vi "UE9 Multiple AIN and Multiple LabJack Loop Example.vi"() -> ()   [LabVIEW 2021]
panel:
  in  "stop":bool
  in  "Ranges B":string[](array[string])=["LJ_rgBIP5V", "LJ_rgBIP5V"]
  in  "Channels B":i32[](array[numeric])=[0, 1]
  out "Values Read B":dbl[](array[numeric]) format="%.6f"
  in  "Address B":string="3"
  in  "ConnectionType":string="LJ_ctUSB"
  in  "Address A":string="2"
  in  "Ranges A":string[](array[string])=["LJ_rgBIP5V", "LJ_rgBIP5V"]
  in  "Channels A":i32[](array[numeric])=[0, 1]
  out "Values Read A":dbl[](array[numeric]) format="%.6f"
  out "Error Message":string
  in  "Resolution":i32=17
  in  "error in":errorcluster
  out "error out":errorcluster
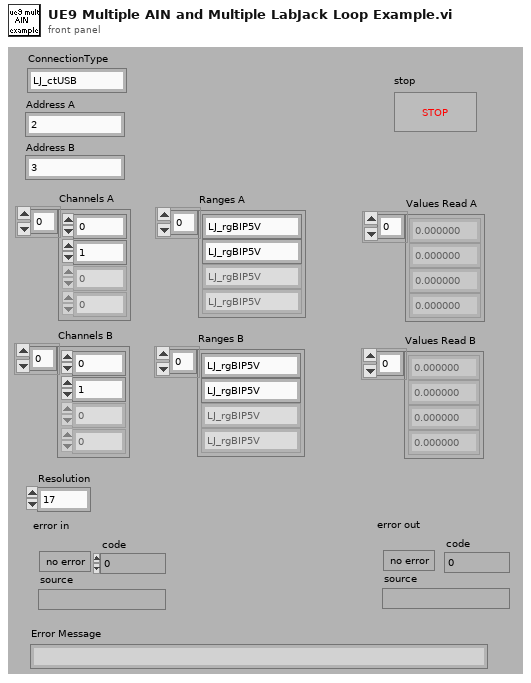
[diagram p1: front panel]
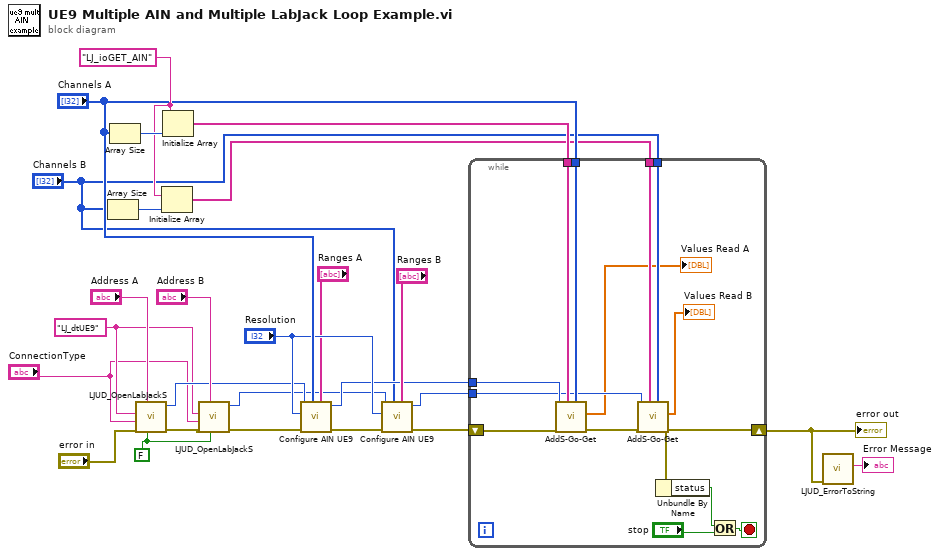
[diagram p0: block diagram]
diagram:
  w2 = "LJ_dtUE9"
  w21 = "LJ_ioGET_AIN" ("IOType")
  w7 = FALSE ("FirstFound")
  n1 = Array Size(array="Channels B") -> (size(s)=w22:i32)
  n2 = Array Size(array="Channels A") -> (size(s)=w23:i32)
  n3 = call "LJUD_OpenLabJackS.vi"("FirstFound"=w7, "Address"="Address A", "error in"="error in", "ConnectionType"="ConnectionType", "DeviceType"=w2) -> ("error out"=w6:errorcluster, "Handle"=w4:i32)  [unwired: 4 in, 1 out]
  n4 = Initialize Array(w21, w22) -> (w11:string[])
  n5 = Initialize Array(w21, w23) -> (w24:string[])
  n6 = call "LJUD_OpenLabJackS.vi"("FirstFound"=w7, "Address"="Address B", "error in"=w6, "ConnectionType"="ConnectionType", "DeviceType"=w2) -> ("error out"=w5:errorcluster, "Handle"=w3:i32)  [unwired: 4 in, 1 out]
  n7 = call "Configure AIN UE9.vi"("Ranges"="Ranges A", "Channels"="Channels A", "error in"=w5, "Resolution"="Resolution", "Handle In"=w4) -> ("error out"=w16:errorcluster, "Handle Out"=w14:i32)  [unwired: 5 in]
  n8 = call "Configure AIN UE9.vi"("Ranges"="Ranges B", "Channels"="Channels B", "error in"=w16, "Resolution"="Resolution", "Handle In"=w3) -> ("error out"=w15:errorcluster, "Handle Out"=w13:i32)  [unwired: 5 in]
  n9 = while {
    tunnel: w11 -> [w32]
    tunnel: "Channels B" -> [w33]
    tunnel: w13 -> [w34]
    tunnel: w14 -> [w35]
    shift-left: w15 -> [w38]
    shift-right: [w36] -> w10
    tunnel: "Channels A" -> [w39]
    tunnel: w24 -> [w40]
    stop <- w29 stop-if-true
    n10 = call "AddS-Go-Get.vi"("Channels"=w39, "IOTypes"=w40, "error in"=w38, "Handle In"=w35) -> ("error out"=w37:errorcluster, "Values Read"=→"Values Read A":dbl[])  [unwired: 5 in, 1 out]
    n11 = call "AddS-Go-Get.vi"("Channels"=w33, "IOTypes"=w32, "error in"=w37, "Handle In"=w34) -> ("error out"=w36:errorcluster, "Values Read"=→"Values Read B":dbl[])  [unwired: 5 in, 1 out]
    n12 = Unbundle By Name(w36) -> ("status"=w27:bool)
    n13 = Or(x=w27, y="stop") -> (x .or. y?=w29:bool)
  }
  "error out" <- w10
  n14 = call "LJUD_ErrorToString.vi"("error in"=w10) -> ("String"=→"Error Message":string)  [unwired: 10 in]
